vi "zmq_close.vi"(3 "error in":errorcluster, 5 "socket":refnum<class "zmq_socket.lvclass">) -> (0 "error out":errorcluster)   [LabVIEW 2010, in "zeromq.lvlib" / "zmq_socket.lvclass"]
doc: "Signal that the socket is no longer required and to free it once pending operations are finished.\n\nNote that this is a <b>non-blocking</b> function and the socket is not necessarily closed when it returns. Any operations pending will be completed before the socket is closed and port freed. To interrupt blocking calls use ctx_destroy.\n\nDetailed API documentation: http://api.zeromq.org/3-2:zmq-close"
uses:
  zmq_socket.lvclass
  zmq_socket.lvclass/zmq_socket.ctl
  <vilib>/Utility/error.llb/Error Cluster From Error Code.vi
  zeromq.lvlib
panel:
  # "ØMQ"
  # "labview"
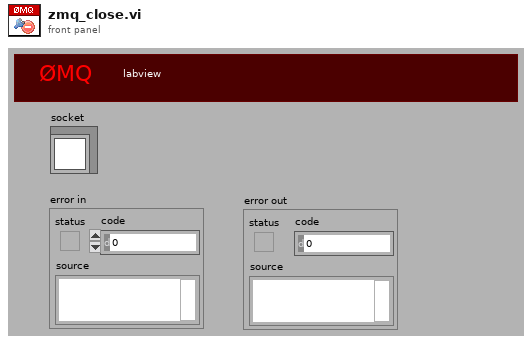
[diagram p1: front panel]
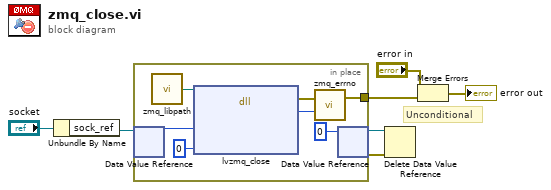
[diagram p0: block diagram]
diagram:
  # "Unconditional"
  n1 = Unbundle By Name("socket") -> ("sock_ref"=w6:refnum<data-value>)
  n2 = in-place {
    in-place-border: [w12] -> w2
    n3 = in-place-dvr #1(w6) -> (w10:u64)  [unwired: 1 out]
    n4 = call "zmq_libpath.vi"() -> ("path"=w8:path)
    n5 = dll-call lib="?" fn="lvzmq_close" ("libzmq.dll:zmq_close")(path in=w8, "sock_obj"=w10, "flags"=0 ("kill")) -> (error out=w13:errorcluster, "return"=w14:i32)  [unwired: 4 in, 1 out]
    n6 = call "zmq_errno.vi"("retval"=w14, "error in"=w13) -> ("error out"=w12:errorcluster)  [unwired: 1 out]
    n7 = in-place-dvr #1(u64 0 ("data value")) -> (w4:refnum<data-value>, w5:errorcluster)
  }
  n8 = Delete Data Value Reference(data value reference=w4, error in=w5) -> ()  [unwired: 2 out]
  n9 = Merge Errors("error in", w2) -> (→"error out":errorcluster)
